vi "Distance Drive.vi"(8 "Distance":dbl, 9 "Location":dbl) -> ()   [LabVIEW 2014]
uses:
  <vilib>/Rock Robotics/WPI/RobotDrive/WPI_RobotDriveGetSetRefNum.vi
  <vilib>/Rock Robotics/WPI/RobotDrive/WPI_RobotDriveMecanumDrive_Cartesian.vi
  Robot Global Data.vi
panel:
  out "Drive Speed":dbl
  in  "Drive Gain":dbl=0.01 step=0.0025
  in  "desired heading":dbl
  in  "multiplication control":dbl=0.1 format="%#_13g"
  out "drive strength":dbl
  in  "X":dbl format="%#_13g"
  out "Angle":dbl
  out "Angular Rate":dbl
  out "Move":bool
  in  "Gyro Reset":bool
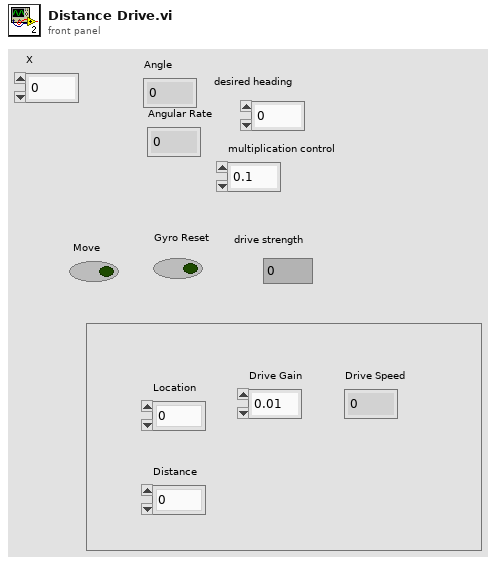
[diagram p1: front panel]
types:
  T1 = typedef "WPI_GyroDevRef.ctl" = cluster{"DevStatus":errorcluster, "Analog Module":T2, "Analog Channel":T3, "Offset":dbl, "Gain (VoltsPerDegree/Second)":dbl}
  T2 = typedef "FPGA_TypedefAnalogModule.ctl" = enum16{"Controller 1"}
  T3 = typedef "FPGA_AIChannel.ctl" = enum8{"AI 0", "AI 1", "AI 2", "AI 3", "AI MXP 0", "AI MXP 1", "AI MXP 2", "AI MXP 3", "Invalid"}
  T4 = typedef "WPI_RobotDriveDevRef.ctl" = cluster{"DevStatus":errorcluster, "Motors[]":T5[], "Square Inputs":bool, "Max Output":dbl}
  T5 = typedef "WPI_MotorControlDeviceRef.ctl" = cluster{"DeviceStatus":errorcluster, "Type":T6, "PWM":cluster{"Controller":T7, "PWM Channel":T8, "DeadBand":T9}, "CAN":cluster{"Device Number":u8, "Control Mode":T10, "Semaphore":T11, "Max Vout":dbl, "TalonSRX Control Mode":T12}, "Invert":bool, "TransformRef":T13, "InvTransformRef":T13}
  T6 = typedef "WPI_MotorControlType.ctl" = enum16{"PWM", "CAN", "CANTalonSRX"}
  T7 = typedef "FPGA_TypedefDigitalModule.ctl" = enum16{"Controller 1"}
  T8 = typedef "FPGA_DIOPWMChannel.ctl" = enum8{"PWM 0", "PWM 1", "PWM 2", "PWM 3", "PWM 4", "PWM 5", "PWM 6", "PWM 7", "PWM 8", "PWM 9", "PWM MXP 0", "PWM MXP 1", "PWM MXP 2", "PWM MXP 3", "PWM MXP 4", "PWM MXP 5", "PWM MXP 6", "PWM MXP 7", "PWM MXP 8", "PWM MXP 9", "Invalid"}
  T9 = typedef "WPI_PWMDeadband.ctl" = cluster{"Name":string, "maxPositivePwm":i32, "minPositivePwm":i32, "centerPwm":i32, "maxNegativePwm":i32, "minNegativePwm":i32, "angularRange":u16}
  T10 = typedef "WPI_CANJaguar_ControlMode.ctl" = enum8{"Percent VBus", "Current", "Speed", "Position", "Voltage"}
  T11 = typedef "Semaphore RefNum" = refnum<k1>
  T12 = typedef "WPI_CANTalonSRX_APIControlMode.ctl" = enum8{"Percent VBus", "Speed", "Position", "Slave", "Unchanged / Invalid"}
  T13 = typedef "WPI_PWMTransform_ConPane.ctl" = refnum<vi>
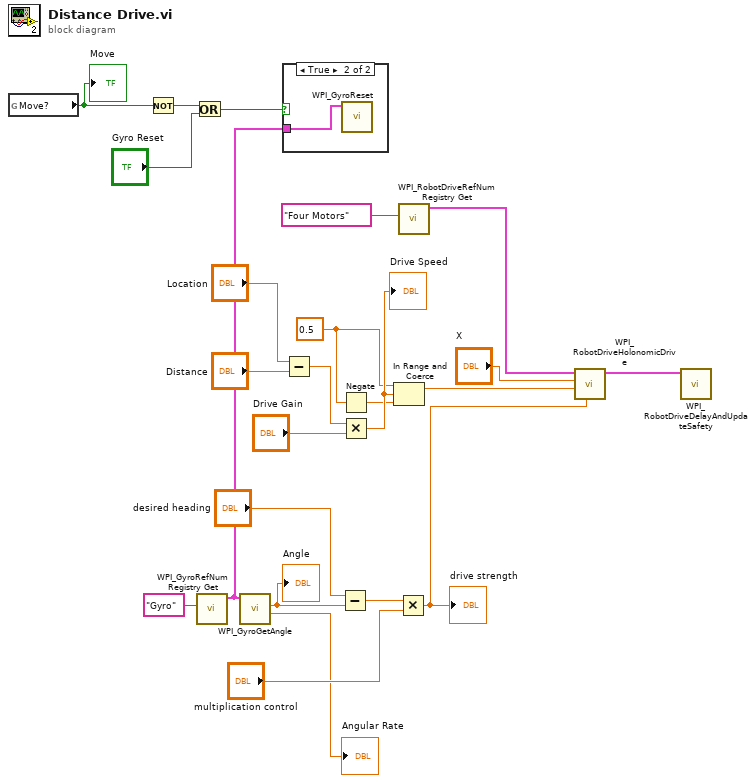
[diagram p0: block diagram]
diagram:
  w14 = 0.5 ("upper limit")
  n1 = global read "Robot Global Data.vi" "Move?"() -> (w11:bool)
  "Move" <- w11
  n2 = Not(x=w11) -> (.not. x?=w21:bool)
  n3 = Or(x=w21, y="Gyro Reset") -> (x .or. y?=w22:bool)
  n4 = call <vilib>:"WPI_GyroRefNum Registry Get.vi"("refnum name"="Gyro") -> ("GyroDevRef"=w20:T1)  [unwired: 9 in, 1 out]
  n5 = call <vilib>:"WPI_GyroGetAngle.vi"("GyroDevRef"=w20) -> ("Angular Rate"=→"Angular Rate":dbl, "Angle"=w1:dbl)  [unwired: 7 in, 2 out]
  "Angle" <- w1
  n6 = case shown="True" w22 {
    tunnel: w20 -> [_ w25]
    frame False {
    }
    frame True {
      n7 = call <vilib>:"WPI_GyroReset.vi"("GyroDevRef"=w25) -> ()  [unwired: 9 in, 2 out]
    }
  }
  n8 = Subtract(x="Location", y="Distance") -> (x-y=w17:dbl)
  n9 = Subtract(x="desired heading", y=w1) -> (x-y=w9:dbl)
  n10 = Negate(x=w14) -> (-x=w13:dbl)
  n11 = Multiply(x=w17, y="Drive Gain") -> (x*y=w15:dbl)
  "Drive Speed" <- w15
  n12 = In Range and Coerce(upper limit=w14, x=w15, lower limit=w13) -> (coerced(x)=w12:dbl)  [unwired: 1 out]
  n13 = Multiply(x=w9, y="multiplication control") -> (x*y=w10:dbl)
  "drive strength" <- w10
  n14 = call <vilib>:"WPI_RobotDriveRefNum Registry Get.vi"("refnum name"="Four Motors") -> ("RobotDriveDevRef"=w5:T4)  [unwired: 1 in, 9 out]
  n15 = call-poly <vilib>:"WPI_RobotDriveHolonomicDrive.vi"("Rotation"=w10, "Y"=w12, "X"="X", "RobotDriveDevRef"=w5) -> ("RobotDriveDevRef"=w4:T4)  [unwired: 5 in, 2 out]
  n16 = call <vilib>:"WPI_RobotDriveDelayAndUpdateSafety.vi"("RobotDriveDevRef"=w4) -> ()  [unwired: 9 in, 2 out]
